vi "GetTBS2000.vi"(11 "object in":refnum<class "Application.lvclass">) -> (1 "TBS2000Series":refnum<class "TBS2000Series.lvclass">, 3 "object out":refnum<class "Application.lvclass">)   [LabVIEW 2023, in "Application.lvclass"]
uses:
  Application.lvclass
  Application.lvclass/Application.ctl
  TBS2000Series_class/TBS2000Series.lvclass
panel:
  out "error out":errorcluster
  in  "error in (no error)":errorcluster
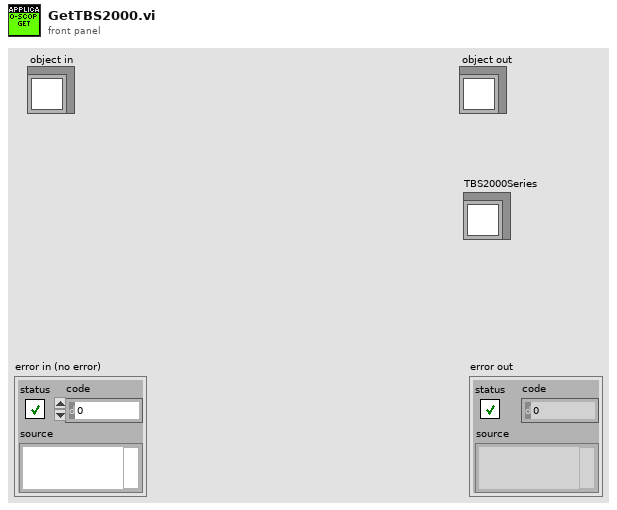
[diagram p1: front panel]
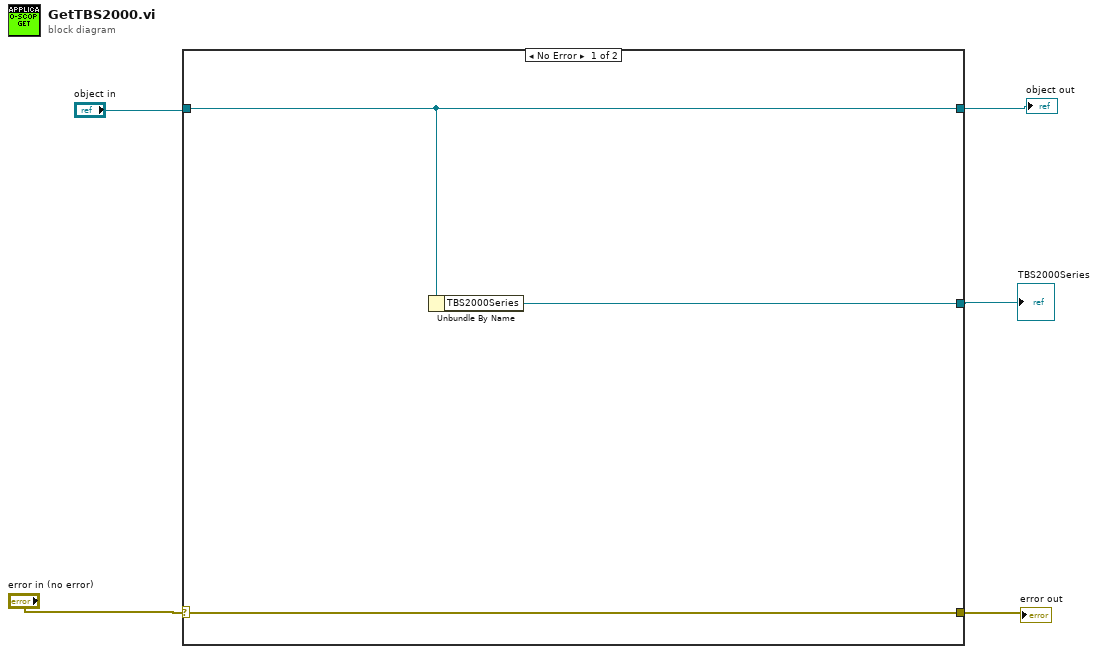
[diagram p0: block diagram]
diagram:
  n1 = case shown="No Error" "error in (no error)" {
    selector: "error in (no error)" -> [w7 w10]
    tunnel: [w7 w10] -> w5
    tunnel: [w6 w9] -> w2
    tunnel: "object in" -> [w6 w9]
    tunnel: [w8 _] -> w1
    frame No Error {
      n2 = Unbundle By Name(w6) -> ("TBS2000Series"=w8:refnum<class "TBS2000Series.lvclass">)
    }
    frame Error {
    }
  }
  "error out" <- w5
  "object out" <- w2
  "TBS2000Series" <- w1
